vi "writedacsettings.vi"(0 "red":bool, 1 "Path":path, 2 "?":T1, 5 "error in (no error)":errorcluster) -> (6 "Path 2":path, 8 "error out":errorcluster)   [LabVIEW 2012]
uses:
  <vilib>/Utility/config.llb/Write Key (Double).vi
  <vilib>/Utility/config.llb/NI_LVConfig.lvlib
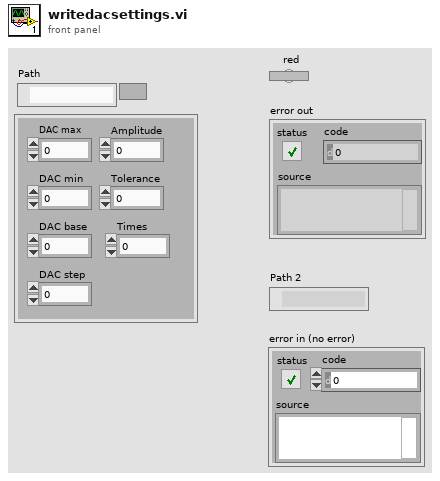
[diagram p1: front panel]
types:
  T1 = cluster{"DAC max":dbl, "DAC min":dbl, "DAC base":dbl, "DAC step":dbl, "Amplitude":dbl, "Tolerance":dbl, "Times":dbl}
  T2 = typedef "NI_LVConfig.lvlib/Config Data RefNum.ctl" = refnum<k1>
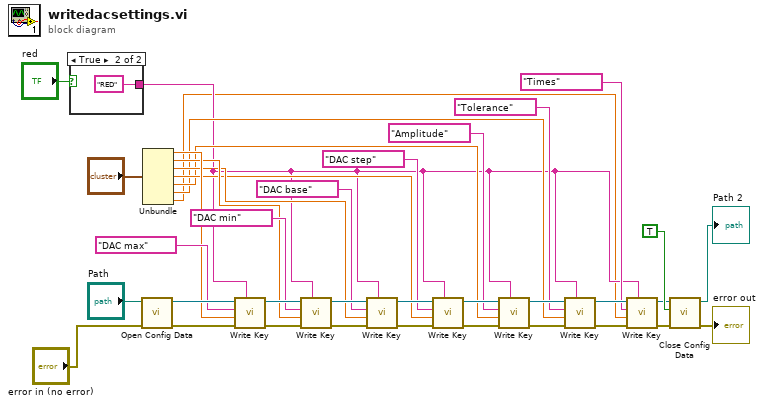
[diagram p0: block diagram]
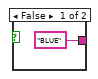
[diagram p2: hidden frame]
diagram:
  n1 = case shown="True" "red" {
    tunnel: ["BLUE" "RED"] -> w3
    frame False {
    }
    frame True {
    }
  }
  n2 = call <vilib>:"Open Config Data.vi"("error in (no error)"="error in (no error)", "configuration file path"="Path") -> ("error out"=w31:errorcluster, "refnum"=w37:T2)  [unwired: 7 in, 1 out]
  n3 = Unbundle("?") -> ("DAC max"=w16:dbl, "DAC min"=w15:dbl, "DAC base"=w14:dbl, "DAC step"=w13:dbl, "Amplitude"=w12:dbl, "Tolerance"=w11:dbl, "Times"=w2:dbl)
  n4 = call-poly <vilib>:"Write Key.vi"("section"=w3, "error in (no error)"=w31, "value"=w16, "key"="DAC max", "refnum"=w37) -> ("error out"=w30:errorcluster, "refnum out"=w36:T2)  [unwired: 4 in, 1 out]
  n5 = call-poly <vilib>:"Write Key.vi"("section"=w3, "error in (no error)"=w30, "value"=w15, "key"="DAC min", "refnum"=w36) -> ("error out"=w29:errorcluster, "refnum out"=w35:T2)  [unwired: 4 in, 1 out]
  n6 = call-poly <vilib>:"Write Key.vi"("section"=w3, "error in (no error)"=w29, "value"=w14, "key"="DAC base", "refnum"=w35) -> ("error out"=w28:errorcluster, "refnum out"=w34:T2)  [unwired: 4 in, 1 out]
  n7 = call-poly <vilib>:"Write Key.vi"("section"=w3, "error in (no error)"=w28, "value"=w13, "key"="DAC step", "refnum"=w34) -> ("error out"=w27:errorcluster, "refnum out"=w33:T2)  [unwired: 4 in, 1 out]
  n8 = call-poly <vilib>:"Write Key.vi"("section"=w3, "error in (no error)"=w27, "value"=w12, "key"="Amplitude", "refnum"=w33) -> ("error out"=w26:errorcluster, "refnum out"=w32:T2)  [unwired: 4 in, 1 out]
  n9 = call-poly <vilib>:"Write Key.vi"("section"=w3, "error in (no error)"=w26, "value"=w11, "key"="Tolerance", "refnum"=w32) -> ("error out"=w7:errorcluster, "refnum out"=w8:T2)  [unwired: 4 in, 1 out]
  n10 = call-poly <vilib>:"Write Key.vi"("section"=w3, "error in (no error)"=w7, "value"=w2, "key"="Times", "refnum"=w8) -> ("error out"=w5:errorcluster, "refnum out"=w6:T2)  [unwired: 4 in, 1 out]
  n11 = call <vilib>:"Close Config Data.vi"("error in (no error)"=w5, "write file if changed (T)"=TRUE, "refnum"=w6) -> ("error out"=→"error out":errorcluster, "file path"=→"Path 2":path)  [unwired: 7 in]
